vi "controlAQuadBOut.vi"(7 "Set":bool, 8 "error in":errorcluster, 9 "ABout in":bool=TRUE, 10 "axis in":u8, 11 "connection ID":refnum<k5>) -> (0 "error out":errorcluster, 1 "ABout out":bool=TRUE, 2 "axis out":u8, 3 "connection ID":refnum<k5>)   [LabVIEW 2016]
panel:
  in  "Set Command":string="com.attocube.amc.rtout.setControlAQuadBOut"
  in  "Get Command":string="com.attocube.amc.rtout.getControlAQuadBOut"
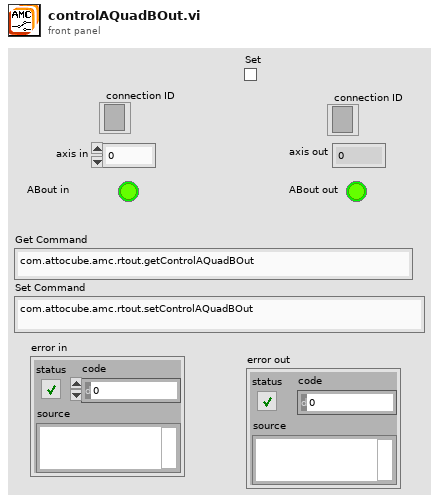
[diagram p1: front panel]
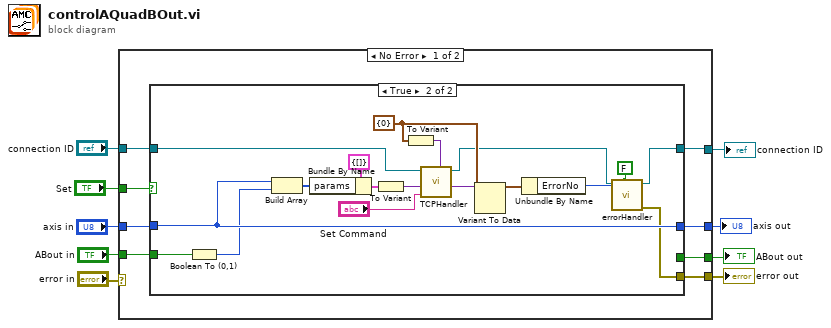
[diagram p0: block diagram]
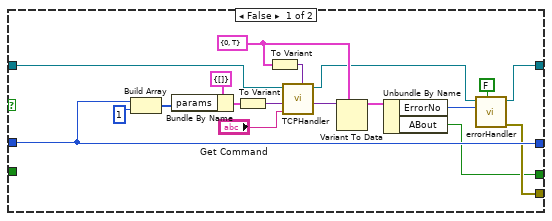
[diagram p2: hidden frame]
diagram:
  n1 = case shown="No Error" "error in" {
    selector: "error in" -> [_ w57]
    tunnel: "axis in" -> [w15 w55]
    tunnel: [w11 w57] -> w8
    tunnel: [w14 w55] -> w7
    tunnel: "Set" -> [w10 _]
    tunnel: "ABout in" -> [w13 w56]
    tunnel: [w16 w54] -> w4
    tunnel: "connection ID" -> [w17 w54]
    tunnel: [w12 w56] -> w2
    frame No Error {
      n2 = case shown="True" w10 {
        tunnel: [w18 w36] -> w16
        tunnel: w17 -> [w25 w48]
        tunnel: w15 -> [w27 w46]
        tunnel: [w27 w46] -> w14
        tunnel: [w24 _] -> w12
        tunnel: [w26 w43] -> w11
        tunnel: w13 -> [_ w38]
        frame False {
          w22 = cluster{"ErrorNo":i16, "ABout":bool} {"ErrorNo"=0, "ABout"=TRUE} ("input cluster")
          n3 = Build Array(w27, 1) -> (w31:i32[])
          n4 = Bundle By Name(cluster=cluster{"params":i16[]} {"params"=[]} ("input cluster"), "params"=w31) -> (w32:cluster{"params":i16[]})
          n5 = To Variant(anything=w32) -> (Variant=w33:variant)
          n6 = To Variant(anything=w22) -> (Variant=w23:variant)
          n7 = call "TCPHandler.vi"("result Types"=w23, "method"="Get Command", "params"=w33, "connection ID"=w25) -> ("result"=w29:variant, "connection ID"=w19:refnum<k5>)  [unwired: 5 in, 1 out]
          n8 = Variant To Data(type=w22, Variant=w29) -> (data=w34:cluster{"ErrorNo":i16, "ABout":bool})  [unwired: 1 in, 1 out]
          n9 = Unbundle By Name(w34) -> ("ErrorNo"=w35:i16, "ABout"=w24:bool)
          n10 = call "errorHandler.vi"("show popup"=FALSE, "error number"=w35, "connection ID"=w19) -> ("error out"=w26:errorcluster, "connection ID"=w18:refnum<k5>)  [unwired: 7 in]
        }
        frame True {
          w41 = cluster{"ErrorNo":i16} {"ErrorNo"=0} ("input cluster")
          n11 = Boolean To (0,1)(Boolean=w38) -> (0, 1=w39:i16)
          n12 = Build Array(w46, w39) -> (w50:i16[])
          n13 = Bundle By Name(cluster=cluster{"params":i64[]} {"params"=[]} ("input cluster"), "params"=w50) -> (w49:cluster{"params":i64[]})
          n14 = To Variant(anything=w49) -> (Variant=w47:variant)
          n15 = To Variant(anything=w41) -> (Variant=w42:variant)
          n16 = call "TCPHandler.vi"("result Types"=w42, "method"="Set Command", "params"=w47, "connection ID"=w48) -> ("result"=w52:variant, "connection ID"=w37:refnum<k5>)  [unwired: 5 in, 1 out]
          n17 = Variant To Data(type=w41, Variant=w52) -> (data=w45:cluster{"ErrorNo":i16})  [unwired: 1 in, 1 out]
          n18 = Unbundle By Name(w45) -> ("ErrorNo"=w44:i16)
          n19 = call "errorHandler.vi"("show popup"=FALSE, "error number"=w44, "connection ID"=w37) -> ("error out"=w43:errorcluster, "connection ID"=w36:refnum<k5>)  [unwired: 7 in]
        }
      }
    }
    frame Error {
    }
  }
  "error out" <- w8
  "axis out" <- w7
  "ABout out" <- w2
  "connection ID" <- w4
